vi "element_editor_methane_run.vi"(11 "Break":refnum<vi>) -> ()   [LabVIEW 2019]
uses:
  lib/libSimulationControl/libSimulationControl.lvlib
panel:
  out "spec":path
  # "*******************************************************************\nBiogas Plant Control\n\nAuthor: Paul Zügel\nGCSC-Frankfurt am Main 2020\n\n*******************************************************************"
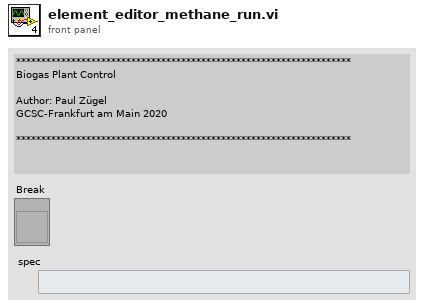
[diagram p1: front panel]
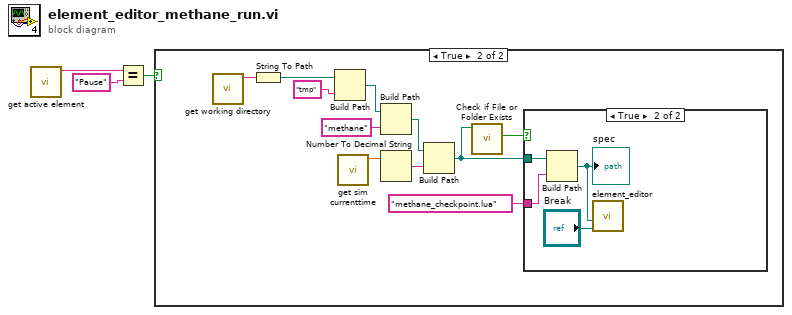
[diagram p0: block diagram]
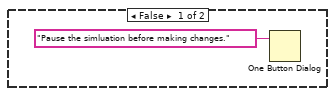
[diagram p2: hidden frame]
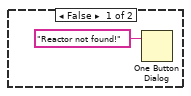
[diagram p3: hidden frame]
diagram:
  n1 = call "get active element.vi"() -> ("active_element"=w3:string)  [unwired: 10 in, 1 out]
  n2 = Equal?(x=w3, y="Pause") -> (x = y?=w1:bool)
  n3 = case shown="True" w1 {
    frame False {
      n4 = One Button Dialog(message="Pause the simluation before making changes.") -> ()  [unwired: 1 in, 1 out]
    }
    frame True {
      n5 = call "get working directory.vi"() -> ("function return"=w9:string)  [unwired: 10 in, 1 out]
      n6 = String To Path(string=w9) -> (path=w10:path)
      n7 = Build Path(base path=w10, name or relative path="tmp") -> (appended path=w11:path)
      n8 = call "get sim currenttime.vi"() -> ("current_time"=w15:dbl)  [unwired: 10 in, 1 out]
      n9 = Build Path(base path=w11, name or relative path="methane") -> (appended path=w14:path)
      n10 = Number To Decimal String(number=w15) -> (decimal integer string=w13:string)  [unwired: 1 in]
      n11 = Build Path(base path=w14, name or relative path=w13) -> (appended path=w6:path)
      n12 = call <vilib>:"Check if File or Folder Exists.vi"("path"=w6) -> ("file or folder exists?"=w8:bool)  [unwired: 8 in, 2 out]
      n13 = case shown="True" w8 {
        tunnel: "methane_checkpoint.lua" ("name or relative path") -> [_ w18]
        tunnel: w6 -> [_ w17]
        frame False {
          n14 = One Button Dialog(message="Reactor not found!") -> ()  [unwired: 1 in, 1 out]
        }
        frame True {
          n15 = Build Path(base path=w17, name or relative path=w18) -> (appended path=w19:path)
          "spec" <- w19
          n16 = call "element_editor.vi"("Break"="Break", "LUA Specification File"=w19) -> ()  [unwired: 5 in, 1 out]
        }
      }
    }
  }
